vi "DSF.Memory.Pointer.Channel Properties.New.vi"(8 "error in (no error)":errorcluster, 11 "count (1)":u64=1 format="%d elements") -> (0 "error out":errorcluster, 3 "Channel Properties pointer":refnum<class "DSF.Memory.Pointer.Channel Properties.lvclass">)   [LabVIEW 2016, in "DSF.Memory.lvlib" / "DSF.Memory.Pointer.Channel Properties.lvclass"]
uses:
  DSF.Memory.Pointer.Channel Properties.lvclass
  C:/Git/SourceTree/DSF/Source/Classes/Memory.Pointer.Array/DSF.Memory.Pointer.Array.lvclass
  Typedefs/DSF.Common.Channel Configuration.ctl
  Typedefs/DSF.Common.DataType.ctl
  DSF.Common.lvlib
  Memory.Pointer.Array/DSF.Memory.Pointer.Array.lvclass
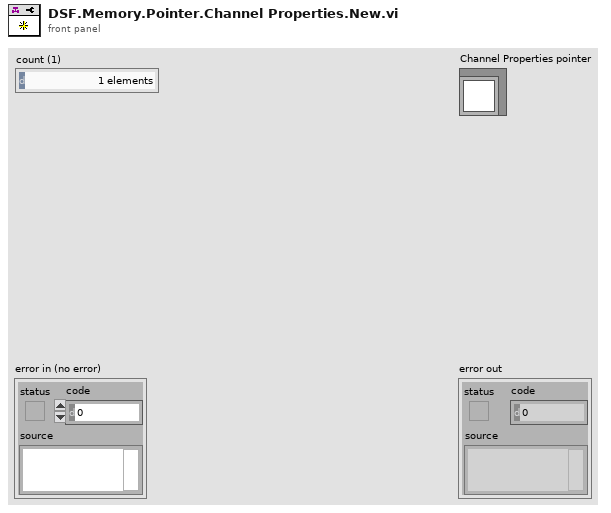
[diagram p1: front panel]
types:
  T1 = typedef "DSF.Common.lvlib/DSF.Common.Channel Configuration.ctl" = cluster{"data type":T2, "offset":u64, "size":u64, "count":u64}
  T2 = typedef "DSF.Common.lvlib/DSF.Common.DataType.ctl" = enum8{"Boolean", "Single", "Double", "Int8", "Int16", "Int32", "Int64", "UInt8", "UInt16", "UInt32", "UInt64"}
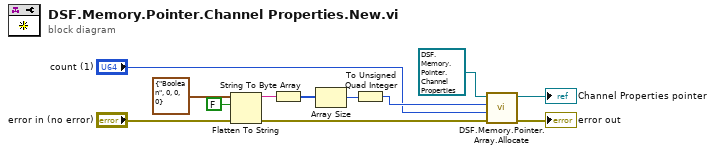
[diagram p0: block diagram]
diagram:
  n1 = Flatten To String(anything=T1 {"data type"=enum."Boolean", "offset"=0, "size"=0, "count"=0} ("Channel properties"), prepend array or string size? (T)=FALSE, error in (no error)="error in (no error)") -> (data string=w9:string, error out=w6:errorcluster)  [unwired: 1 in, 1 out]
  n2 = String To Byte Array(string=w9) -> (unsigned byte array=w8:u8[])
  n3 = Array Size(array=w8) -> (size(s)=w7:i32)
  n4 = To Unsigned Quad Integer(1:w7) -> (0:w5:u64)
  n5 = call "DSF.Memory.Pointer.Array.Allocate.vi"("error in (no error)"=w6, "count (1)"="count (1)", "element size"=w5, "Array Pointer in"=refnum<class "DSF.Memory.Pointer.Channel Properties.lvclass"> refnum ("Channel Properties pointer")) -> ("error out"=→"error out":errorcluster, "Array Pointer out"=→"Channel Properties pointer":refnum<class "DSF.Memory.Pointer.Channel Properties.lvclass">)  [unwired: 6 in]
